vi "internalTesting.vi"() -> ()   [LabVIEW 2017, in "BuildWorker Interface.lvlib" / "BuildWorker Controller.lvclass"]
uses:
  BuildWorker Controller.lvclass
  BuildWorker Controller.lvclass/BuildWorker Controller.ctl
  Read diskLetter.vi
  Read PID.vi
panel:
  out "Next Available Disk Letter":string
  out "PIDs":string[](array[string])
  out "PID":string
  out "diskLetter":string
  in  "remove":bool
  in  "kill":bool
  in  "launch":bool
  in  "new":bool
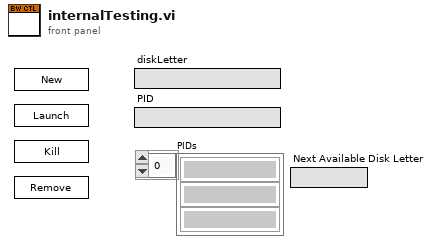
[diagram p1: front panel]
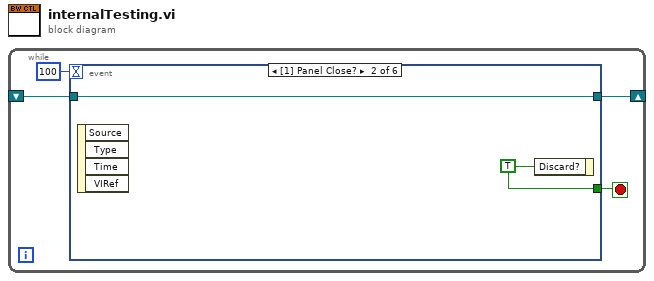
[diagram p0: block diagram]
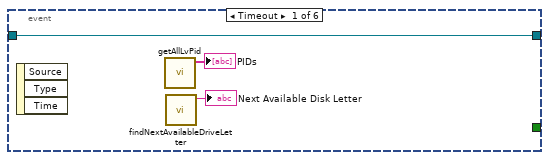
[diagram p2: hidden frame]
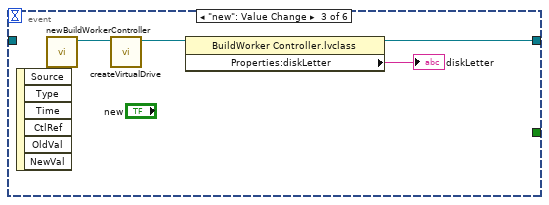
[diagram p3: hidden frame]
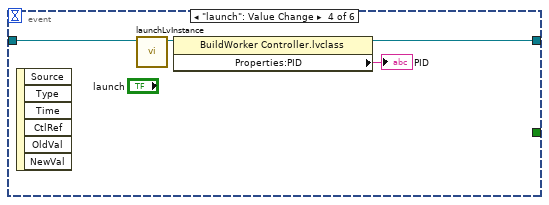
[diagram p4: hidden frame]
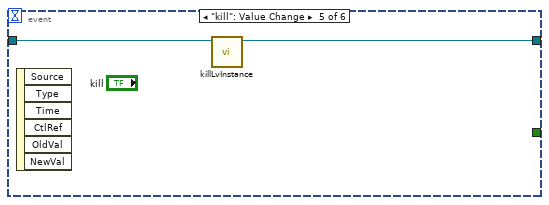
[diagram p5: hidden frame]
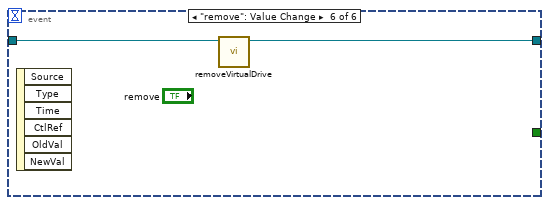
[diagram p6: hidden frame]
diagram:
  n1 = while {
    shift-right: [w3] -> _
    shift-left: _ -> [w2]
    stop <- w4 stop-if-true
    n2 = event shown="[1] Panel Close?" {
      selector: _ -> [_ _ _ _ _ _]
      dyn-events: _ -> [_ _ _ _ _ _]
      timeout: 100 -> [_ _ _ _ _ _]
      tunnel: [_ w9 _ _ _ _] -> w4
      tunnel: [w7 w8 w13 w15 w18 w20] -> w3
      tunnel: w2 -> [w7 w8 _ w17 w19 w21]
      event Timeout {
        n3 = event-data() -> ()  [unwired: 1 in, 3 out]
        n4 = call "getAllLvPid.vi"() -> ("PIDs"=→"PIDs":string[])  [unwired: 10 in, 1 out]
        n5 = call "findNextAvailableDriveLetter.vi"() -> ("Next Available Disk Letter"=→"Next Available Disk Letter":string)  [unwired: 10 in, 1 out]
      }
      event Panel Close? {
        w9 = TRUE ("Discard?")
        n6 = event-data() -> ()  [unwired: 1 in, 4 out]
        n7 = event-data("Discard?"=w9) -> ()  [unwired: 1 in, 1 out]
      }
      event "new": Value Change {
        n8 = event-data() -> ()  [unwired: 1 in, 6 out]
        n9 = call "newBuildWorkerController.vi"() -> ("BuildWorker Controller out"=w11:refnum<class "BuildWorker Controller.lvclass">)  [unwired: 10 in, 1 out]
        n10 = call "createVirtualDrive.vi"("BuildWorker Controller in"=w11) -> ("BuildWorker Controller out"=w10:refnum<class "BuildWorker Controller.lvclass">)  [unwired: 9 in, 1 out]
        n11 = property class="BuildWorker Controller.lvclass"(reference=w10) -> (reference out=w13:refnum<class "BuildWorker Controller.lvclass">, "Properties:diskLetter"=→"diskLetter":string)  [unwired: 1 in, 1 out]
      }
      event "launch": Value Change {
        n12 = event-data() -> ()  [unwired: 1 in, 6 out]
        n13 = call "launchLvInstance.vi"("BuildWorker Controller in"=w17) -> ("BuildWorker Controller out"=w16:refnum<class "BuildWorker Controller.lvclass">)  [unwired: 9 in, 1 out]
        n14 = property class="BuildWorker Controller.lvclass"(reference=w16) -> (reference out=w15:refnum<class "BuildWorker Controller.lvclass">, "Properties:PID"=→"PID":string)  [unwired: 1 in, 1 out]
      }
      event "kill": Value Change {
        n15 = event-data() -> ()  [unwired: 1 in, 6 out]
        n16 = call "killLvInstance.vi"("BuildWorker Controller in"=w19) -> ("BuildWorker Controller out"=w18:refnum<class "BuildWorker Controller.lvclass">)  [unwired: 9 in, 1 out]
      }
      event "remove": Value Change {
        n17 = event-data() -> ()  [unwired: 1 in, 6 out]
        n18 = call "removeVirtualDrive.vi"("BuildWorker Controller in"=w21) -> ("BuildWorker Controller out"=w20:refnum<class "BuildWorker Controller.lvclass">)  [unwired: 9 in, 1 out]
      }
    }
  }
